vi "31 GPS Interrupt RS232 Read (2017).vi"(2 "Comm Port":refnum<visa-resource-name>) -> (5 "GPS Time Code":string, 6 "CPU Time":dbl format="%#.6f", 7 "VISA Error Out":errorcluster)   [LabVIEW 2017]
uses:
  <vilib>/Instr/_visa.llb/VISA Configure Serial Port (Instr).vi
  NI_Timer.dll
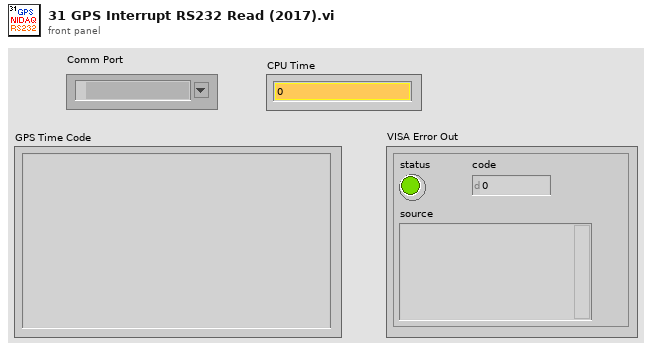
[diagram p1: front panel]
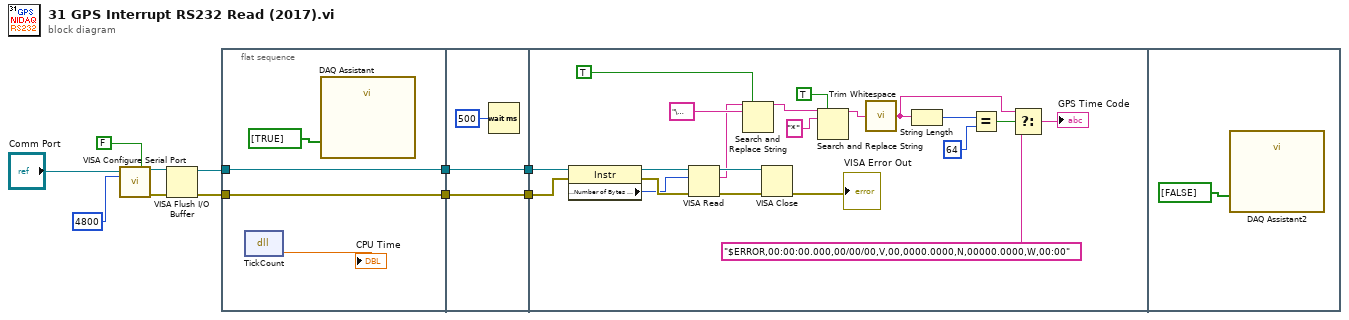
[diagram p0: block diagram]
diagram:
  n1 = call-poly "VISA Configure Serial Port"("VISA resource name"="Comm Port", "Enable Termination\nChar (T)"=FALSE ("Enable Termination\nChar (T)"), "baud rate (9600)"=u32 4800) -> ("VISA resource name out"=w5:refnum<visa-resource-name>, "error out"=w4:errorcluster)  [unwired: 11 in]
  n2 = VISA Flush I/O Buffer(VISA resource name=w5, error in (no error)=w4) -> (VISA resource name out=w2:refnum<visa-resource-name>, error out=w3:errorcluster)  [unwired: 1 in]
  n3 = flat-sequence {
    tunnel: [w15] -> w11
    tunnel: w2 -> [w15]
    tunnel: [w14] -> w10
    tunnel: w3 -> [w14]
    tunnel: [w17] -> w9
    tunnel: w11 -> [w17]
    tunnel: [w16] -> w8
    tunnel: w10 -> [w16]
    tunnel: w9 -> [w39]
    tunnel: w8 -> [w38]
    frame #0 {
      n4 = dll-call lib="C:/Users/willie8/Desktop/Research Summer 2K18/OpenPMU_V1/OpenPMU_V1/SourceCode/OpenPMU-Updated (LabView 2017)/NI_Timer.dll" fn="TickCount"() -> ("return type"=→"CPU Time":dbl)  [unwired: 3 in, 2 out]
      n5 = call "DAQ Assistant"("data"=bool[] [TRUE]) -> ()  [unwired: 17 in, 2 out]
    }
    frame #1 {
      n6 = Wait (ms)(milliseconds to wait=u32 500) -> ()  [unwired: 1 out]
    }
    frame #2 {
      n7 = property class="Instr"(reference=w39, error in=w38) -> (reference out=w37:refnum<visa-resource-name>, error out=w36:errorcluster, "Serial Settings:Number of Bytes at Serial Port"=w33:u32)
      n8 = VISA Read(VISA resource name=w37, byte count=w33, error in (no error)=w36) -> (VISA resource name out=w34:refnum<visa-resource-name>, read buffer=w30:string, error out=w35:errorcluster)  [unwired: 1 out]
      n9 = Search and Replace String(replace all?=TRUE ("replace all? (F)"), input string=w30, search string="\u0000") -> (result string=w27:string)  [unwired: 5 in, 3 out]
      n10 = VISA Close(VISA resource name=w34, error in (no error)=w35) -> (error out=→"VISA Error Out":errorcluster)
      n11 = Search and Replace String(replace all?=TRUE ("replace all? (F)"), input string=w27, search string="*") -> (result string=w26:string)  [unwired: 5 in, 3 out]
      n12 = call <vilib>:"Trim Whitespace.vi"("string"=w26) -> ("trimmed string"=w22:string)  [unwired: 1 in]
      n13 = String Length(string=w22) -> (length=w25:i32)
      n14 = Equal?(x=w25, y=64) -> (x = y?=w23:bool)
      n15 = Select(t=w22, s=w23, f="$ERROR,00:00:00.000,00/00/00,V,00,0000.0000,N,00000.0000,W,00:00") -> (s? t:f=→"GPS Time Code":string)
    }
    frame #3 {
      n16 = call "DAQ Assistant2"("data"=bool[] [FALSE]) -> ()  [unwired: 17 in, 2 out]
    }
  }
